vi "STS Calculator_2014_05_18.vi"(8 "NumPts":i32=3, 10 "Saturation Id":dbl[](array[numeric]), 11 "Vg Column":dbl[](array[numeric])) -> (0 "STS Index":dbl, 1 "NumPts 2":i32=3, 2 "XY Graph":cluster{dbl[], dbl[]}[](graph), 3 "Sub Threshold Swing":dbl, 5 "Used Points":cluster{"Vg Used":dbl[], "Id Used":dbl[]})   [LabVIEW 2012]
uses:
  <vilib>/Analysis/NI_AALPro.lvlib
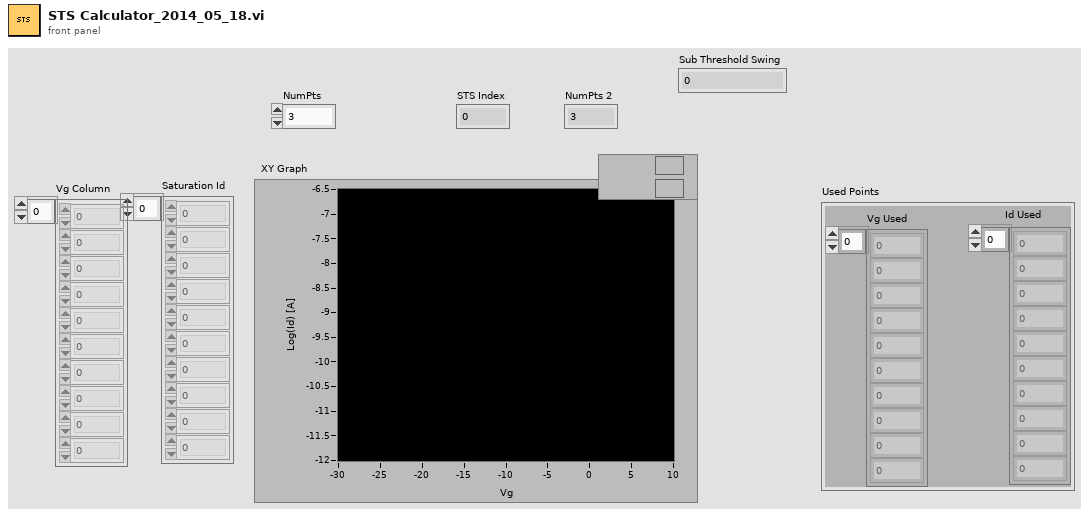
[diagram p1: front panel]
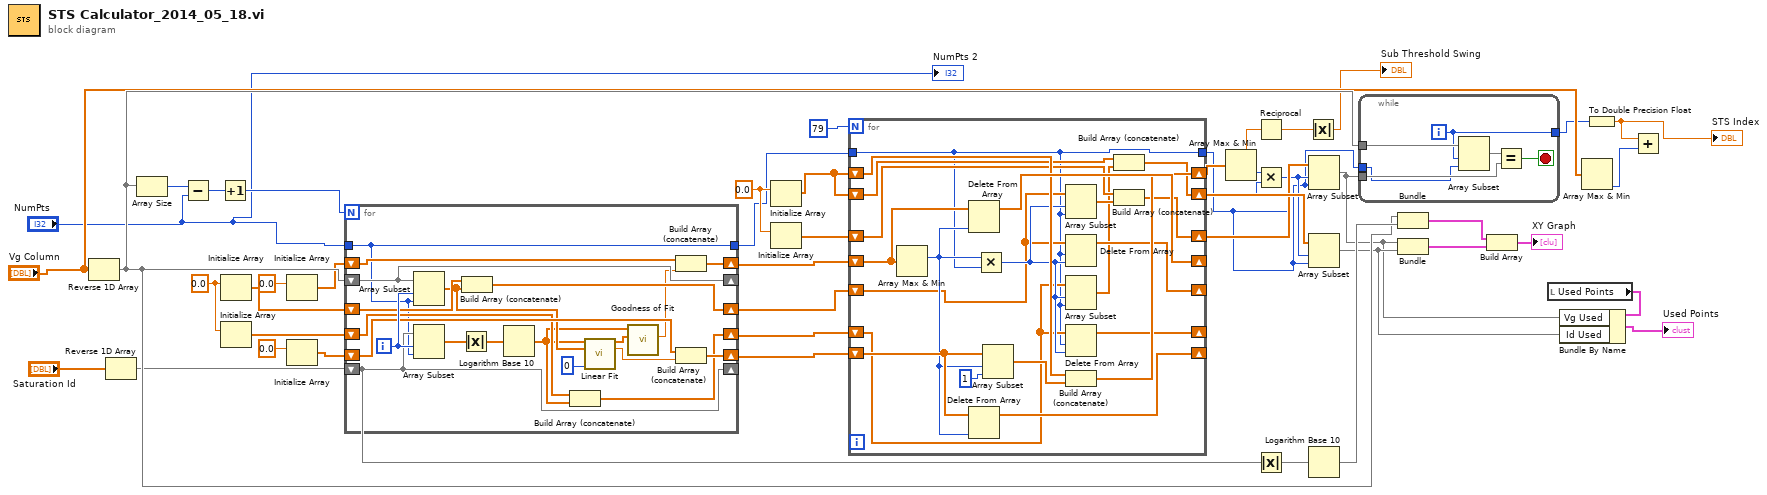
[diagram p0: block diagram]
diagram:
  w23 = 0.0
  w29 = 0.0
  n1 = Reverse 1D Array(array="Vg Column") -> (reversed array=w41:dbl[])
  n2 = Reverse 1D Array(array="Saturation Id") -> (reversed array=w10:dbl[])
  n3 = Array Size(array=w41) -> (size(s)=w40:i32)
  n4 = Subtract(x=w40, y="NumPts") -> (x-y=w16:i32)
  n5 = Increment(x=w16) -> (x+1=w15:i32)
  n6 = Initialize Array(w29) -> (w27:dbl[])  [unwired: 1 in]
  n7 = Initialize Array(w29) -> (w28:dbl[])  [unwired: 1 in]
  n8 = Initialize Array(0.0) -> (w38:dbl[])  [unwired: 1 in]
  n9 = Initialize Array(0.0) -> (w39:dbl[])  [unwired: 1 in]
  n10 = for {
    N: w15 -> [_]
    shift-right: [w53] -> _
    shift-left: w41 -> [w53]
    shift-right: [w59] -> _
    shift-left: w10 -> [w59]
    shift-right: [w63] -> w34
    shift-left: w39 -> [w62]
    shift-right: [w61] -> w32
    shift-left: w38 -> [w60]
    tunnel: "NumPts" -> [w46]
    shift-right: [w56] -> w26
    shift-left: w28 -> [w57]
    shift-right: [w54] -> w25
    shift-left: w27 -> [w55]
    tunnel: [w46] -> w9
    i -> [w65]
    n11 = Array Subset(array=w53, index=w65, length=w46) -> (w52:dbl[])
    n12 = Array Subset(array=w59, index=w65, length=w46) -> (w47:dbl[])
    n13 = Absolute Value(x=w47) -> (abs(x)=w48:dbl[])
    n14 = Build Array (concatenate)(w55, w52) -> (w54:dbl[])
    n15 = Logarithm Base 10(1:w48) -> (0:w49:dbl[])
    n16 = Build Array (concatenate)(w57, w49) -> (w56:dbl[])
    n17 = call <vilib>:"Linear Fit.vi"("Y"=w49, "X"=w52, "method"=0) -> ("Best Linear Fit"=w51:dbl[], "slope"=w64:dbl)  [unwired: 8 in, 3 out]
    n18 = call <vilib>:"Goodness of Fit.vi"("Best Fit"=w51, "Y"=w49) -> ("R-square"=w50:dbl)  [unwired: 6 in, 3 out]
    n19 = Build Array (concatenate)(w60, w50) -> (w61:dbl[])
    n20 = Build Array (concatenate)(w62, w64) -> (w63:dbl[])
  }
  n21 = Initialize Array(w23) -> (w19:dbl[])  [unwired: 1 in]
  n22 = Initialize Array(w23) -> (w24:dbl[])  [unwired: 1 in]
  n23 = for {
    N: 79 -> [_]
    shift-right: [w85] -> _
    shift-left: w32 -> [w86]
    shift-right: [w70] -> _
    shift-left: w34 -> [w71]
    shift-right: [w82] -> w33
    shift-left: w19 -> [w81]
    shift-right: [w80] -> _
    shift-left: w26 -> [w68]
    shift-right: [w78] -> _
    shift-left: w25 -> [w67]
    tunnel: w9 -> [w66]
    shift-right: [w77] -> w22
    shift-left: w19 -> [w76]
    shift-right: [w75] -> w21
    shift-left: w24 -> [w74]
    tunnel: [w66] -> w8
    n24 = Array Max & Min(array=w86) -> (max index (indices)=w69:i32)  [unwired: 3 out]
    n25 = Delete From Array(array=w86, index=w69) -> (array with subset deleted=w85:dbl[])  [unwired: 1 in, 1 out]
    n26 = Delete From Array(array=w71, index=w69) -> (array with subset deleted=w70:dbl[])  [unwired: 1 in, 1 out]
    n27 = Multiply(x=w69, y=w66) -> (x*y=w79:i32)
    n28 = Array Subset(array=w71, index=w69, length=1) -> (w83:dbl[])
    n29 = Array Subset(array=w67, index=w79, length=w66) -> (w73:dbl[])
    n30 = Delete From Array(array=w67, length=w66, index=w79) -> (array with subset deleted=w78:dbl[])  [unwired: 1 out]
    n31 = Array Subset(array=w68, index=w79, length=w66) -> (w72:dbl[])
    n32 = Delete From Array(array=w68, length=w66, index=w79) -> (array with subset deleted=w80:dbl[])  [unwired: 1 out]
    n33 = Build Array (concatenate)(w81, w83) -> (w82:dbl[])
    n34 = Build Array (concatenate)(w76, w72) -> (w77:dbl[])
    n35 = Build Array (concatenate)(w74, w73) -> (w75:dbl[])
  }
  n36 = Array Max & Min(array=w33) -> (min value=w44:dbl, min index (indices)=w20:i32)  [unwired: 2 out]
  n37 = Reciprocal(x=w44) -> (1/x=w45:dbl)
  n38 = Multiply(x=w20, y=w8) -> (x*y=w18:i32)
  n39 = Absolute Value(x=w10) -> (abs(x)=w43:dbl[])
  n40 = Absolute Value(x=w45) -> (abs(x)=→"Sub Threshold Swing":dbl)
  n41 = Array Subset(array=w21, index=w18, length=w8) -> (w12:dbl[])
  n42 = Array Subset(array=w22, index=w18, length=w8) -> (w13:dbl[])
  n43 = Logarithm Base 10(1:w43) -> (0:w42:dbl[])
  n44 = while {
    tunnel: w41 -> [w91]
    tunnel: w12 -> [w90]
    tunnel: [w88] -> w4
    tunnel: w8 -> [w87]
    i -> [w88]
    stop <- w92 stop-if-true
    n45 = Array Subset(array=w91, index=w88, length=w87) -> (w89:dbl[])
    n46 = Equal?(x=w89, y=w90) -> (x = y?=w92:bool)
  }
  n47 = Bundle(w41, w42) -> (w30:cluster{dbl[], dbl[]})  [unwired: 1 in]
  n48 = Bundle(w12, w13) -> (w17:cluster{dbl[], dbl[]})  [unwired: 1 in]
  n49 = Build Array(w30, w17) -> (→"XY Graph":cluster{dbl[], dbl[]}[])
  n50 = local read "Used Points"() -> (w14:cluster{"Vg Used":dbl[], "Id Used":dbl[]})
  n51 = Bundle By Name(cluster=w14, "Vg Used"=w12, "Id Used"=w13) -> (→"Used Points":cluster{"Vg Used":dbl[], "Id Used":dbl[]})
  n52 = Array Max & Min(array="Vg Column") -> (min index (indices)=w3:i32)  [unwired: 3 out]
  n53 = To Double Precision Float(number=w4) -> (double precision float=w2:dbl)
  "STS Index" <- w2
  n54 = Add(x=w2, y=w3) -> ()  [unwired: 1 out]
  "NumPts 2" <- "NumPts"
